vi "Max ESR.vi"(11 "Raw ESR sum":dbl[](array[numeric])) -> (3 "Max ESR":dbl[](array[numeric]))   [LabVIEW 2019, in "Main.lvclass"]
uses:
  Main.lvclass
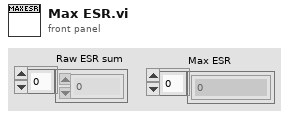
[diagram p1: front panel]
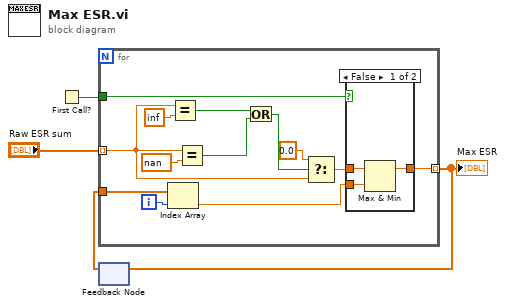
[diagram p0: block diagram]
diagram:
  n1 = First Call?() -> (First Call?: T/F=w2:bool)
  n2 = feedback #1() -> (w3:dbl[])  [unwired: 1 in]
  n3 = for {
    tunnel: "Raw ESR sum" -> [w6] mode=indexing
    tunnel: w3 -> [w15]
    tunnel: [w17] -> w1 mode=indexing
    tunnel: w2 -> [w16]
    i -> [w14]
    n4 = Index Array(array=w15, index=w14) -> (element=w13:dbl)
    n5 = Equal?(x=w6, y=inf) -> (x = y?=w10:bool)
    n6 = Equal?(x=w6, y=nan) -> (x = y?=w9:bool)
    n7 = Or(x=w10, y=w9) -> (x .or. y?=w8:bool)
    n8 = Select(t=0.0, s=w8, f=w6) -> (s? t:f=w5:dbl)
    n9 = case shown="False" w16 {
      tunnel: w5 -> [w20 w21]
      tunnel: w13 -> [w19 _]
      tunnel: [w18 w21] -> w17
      frame False {
        n10 = Max & Min(x=w20, y=w19) -> (max(x,y)=w18:dbl)  [unwired: 1 out]
      }
      frame True {
      }
    }
  }
  "Max ESR" <- w1
  n11 = feedback-in #1(w1) -> ()
